vi "mqttCmdAcknowledge.vi"(0 "_mqtt in":refnum<class "mqttCmdPublish.lvclass">, 11 "error in (no error)":errorcluster) -> (4 "_mqtt out":refnum<class "mqttCmdPublish.lvclass">, 8 "notification":T1, 15 "error out":errorcluster)   [LabVIEW 2017, in "mqttCmdPublish.lvclass"]
uses:
  mqttCmdPublish.lvclass
  K:/Cutting Technology/1 - In scope projects/AI3568 Catapult Programme 2017-18/5 - Software Files/development/mqtt Folder/src/class/mqtt/mqttCmd/mqttCmd.lvclass
  mqttTypedef/mqttRXdataCluster.ctl
  mqttTypedef/mqttFixedHeaderResponse.ctl
  mqttTypedef/mqttQOSlevel.ctl
  mqttTypedef/mqttMessageType.ctl
  mqttCmd.lvclass/mqttCmd.ctl
  mqttCmd.lvclass
panel:
  out "timed out? 2":bool
  out "timed out?":bool
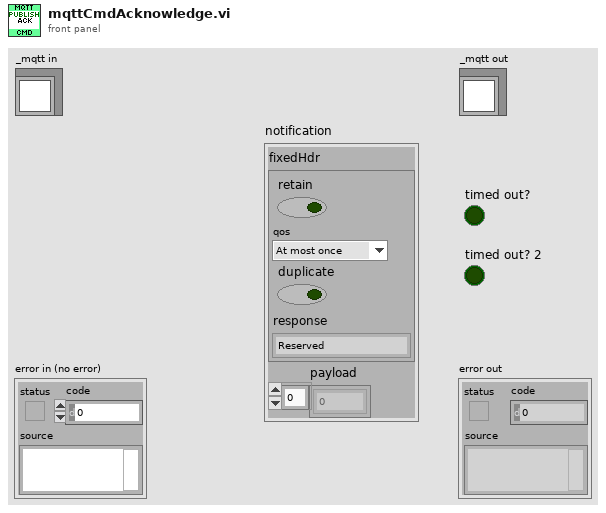
[diagram p1: front panel]
types:
  T1 = typedef "mqttRXdataCluster.ctl" = cluster{"fixedHdr":T2, "payload":u8[]}
  T2 = typedef "mqttFixedHeaderResponse.ctl" = cluster{"retain":bool, "qos":T3, "duplicate":bool, "response":T4}
  T3 = typedef "mqttQOSlevel.ctl" = enum8{"At most once", "At least once", "Exactly once", "Reserved"}
  T4 = typedef "mqttMessageType.ctl" = enum32{"Reserved", "CONNECT", "CONNACK", "PUBLISH", "PUBACK", "PUBREC", "PUBREL", "PUBCOMP", "SUBSCRIBE", "SUBACK", "UNSUBSCRIBE", "UNSUBACK", "PINGREQ", "PINGRESP", "DISCONNECT", "Reserved2"}
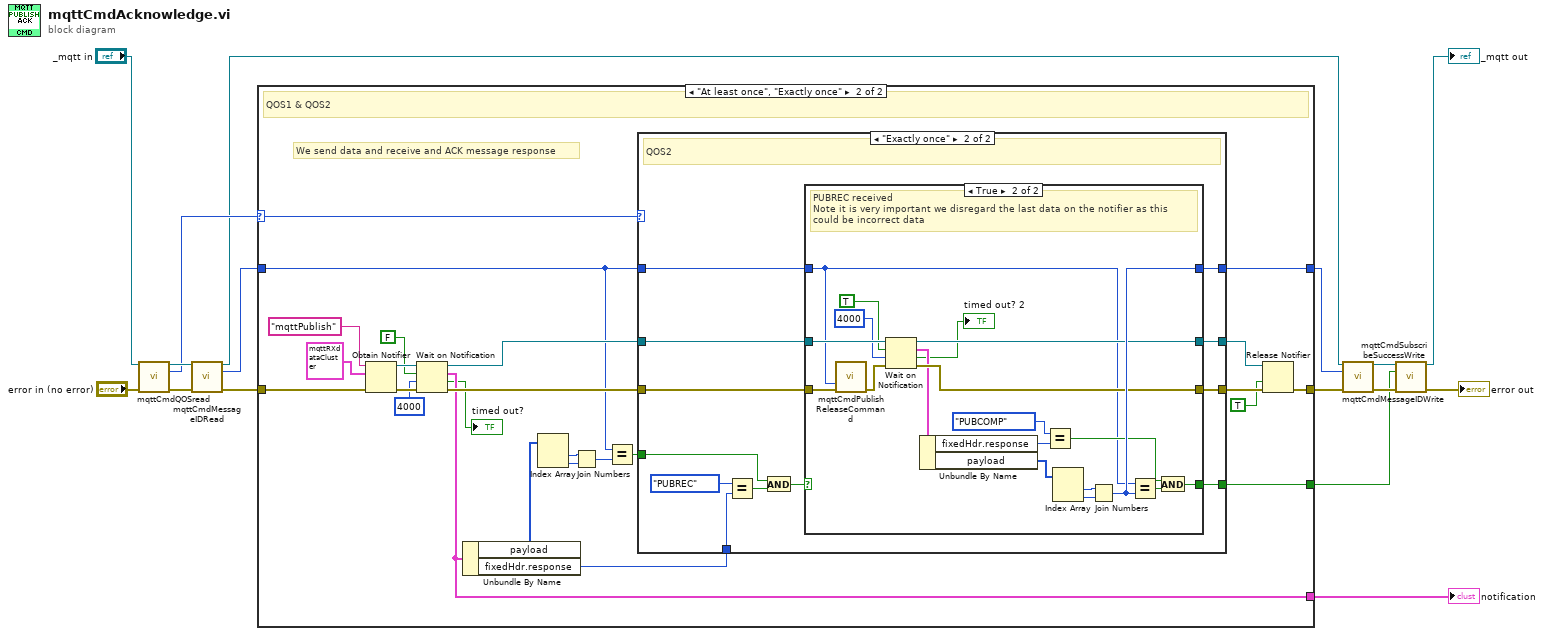
[diagram p0: block diagram]
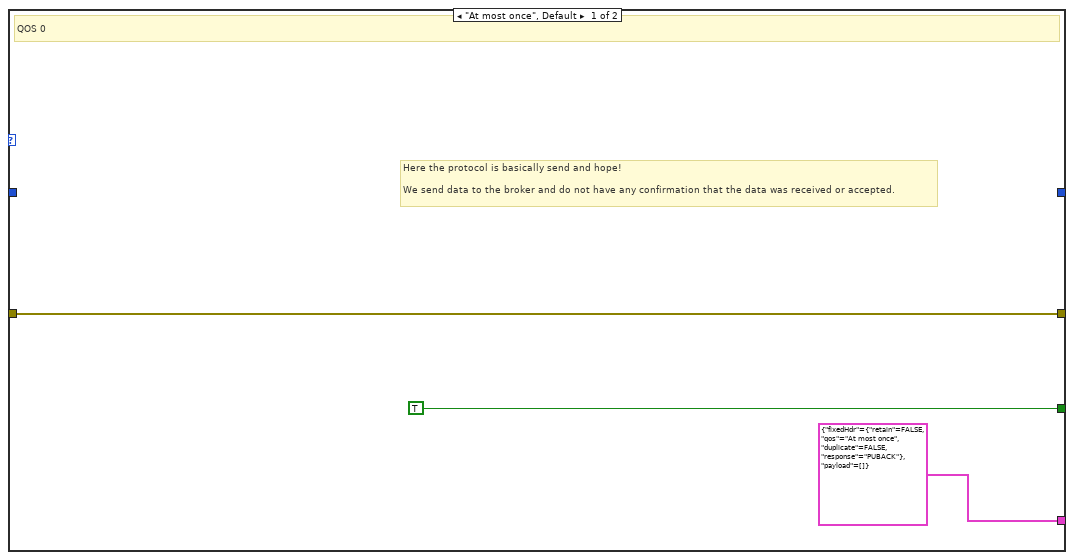
[diagram p2: hidden frame]
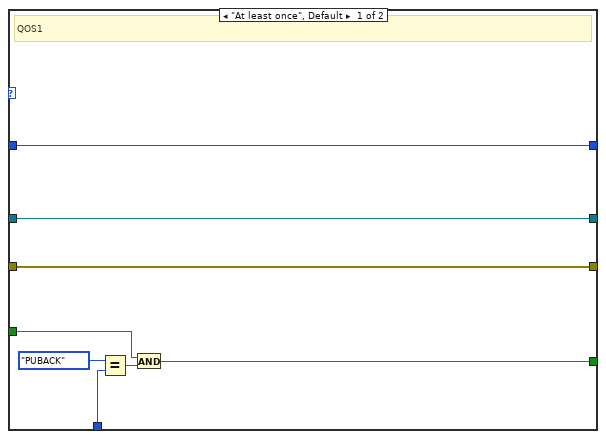
[diagram p3: hidden frame]
diagram:
  n1 = call "mqttCmdQOSread.vi"("mqttBrokerCommand in"="_mqtt in", "error in (no error)"="error in (no error)") -> ("mqttBrokerCommand out"=w14:refnum<class "mqttCmdPublish.lvclass">, "QoS"=w11:T3, "error out"=w15:errorcluster)  [unwired: 11 in]
  n2 = call "mqttCmdMessageIDRead.vi"("mqttBrokerCommand in"=w14, "error in (no error)"=w15) -> ("mqttBrokerCommand out"=w6:refnum<class "mqttCmdPublish.lvclass">, "messageID"=w12:u16, "error out"=w13:errorcluster)  [unwired: 11 in]
  n3 = case shown="\"At least once\", \"Exactly once\"" w11 {
    selector: w11 -> [_ w44]
    tunnel: [w19 w31] -> w9
    tunnel: w13 -> [w19 w38]
    tunnel: [_ w42] -> w8
    tunnel: [TRUE w43] -> w2
    tunnel: w12 -> [_ w25]
    tunnel: [T1 {"fixedHdr"={"retain"=FALSE, "qos"=enum."At most once", "duplicate"=FALSE, "response"=enum."PUBACK"}, "payload"=[]} ("notification") w22] -> w10
    frame "At most once", Default {
      # "Here the protocol is basically send and hope!\n\nWe send data to the broker and do not have any confirmation that the data was received or accepted."
      # "QOS 0"
    }
    frame "At least once", "Exactly once" {
      # "We send data and receive and ACK message response"
      # "QOS1 & QOS2"
      n4 = Obtain Notifier(name (unnamed)="mqttPublish", notification data type=T1 {"fixedHdr"={"retain"=FALSE, "qos"=enum."At most once", "duplicate"=FALSE, "response"=enum."Reserved"}, "payload"=[]} ("notification"), error in (no error)=w38) -> (notifier out=w36:refnum<notifier>, error out=w41:errorcluster)  [unwired: 1 in, 1 out]
      n5 = Wait on Notification(notifier=w36, ignore previous (F)=FALSE, timeout in ms (-1)=4000, error in (no error)=w41) -> (notifier out=w35:refnum<notifier>, notification=w22:T1, timed out?=→"timed out?":bool, error out=w37:errorcluster)
      n6 = Unbundle By Name(w22) -> ("payload"=w27:u8[], "fixedHdr.response"=w23:T4)
      n7 = Index Array(array=w27) -> (element #1=w28:u8, element #2=w29:u8)  [unwired: 2 in]
      n8 = Join Numbers(hi=w28, lo=w29) -> ((hi.lo)=w26:u16)
      n9 = Equal?(x=w25, y=w26) -> (x = y?=w24:bool)
      n10 = case shown="\"Exactly once\"" w44 {
        tunnel: [w45 w62] -> w43
        tunnel: [w52 w64] -> w33
        tunnel: w37 -> [w52 w63]
        tunnel: w25 -> [w48 w54]
        tunnel: [w48 w61] -> w42
        tunnel: w23 -> [w50 w59]
        tunnel: w35 -> [w49 w58]
        tunnel: [w49 w55] -> w34
        tunnel: w24 -> [w47 w53]
        frame "At least once", Default {
          # "QOS1"
          n11 = Equal?(x=mqttMessageType."PUBACK", y=w50) -> (x = y?=w46:bool)
          n12 = And(x=w47, y=w46) -> (x .and. y?=w45:bool)
        }
        frame "Exactly once" {
          # "QOS2"
          n13 = Equal?(x=mqttMessageType."PUBREC", y=w59) -> (x = y?=w57:bool)
          n14 = And(x=w53, y=w57) -> (x .and. y?=w56:bool)
          n15 = case shown="True" w56 {
            selector: w56 -> [w68 _]
            tunnel: [w67 w84] -> w64
            tunnel: w63 -> [w67 w71]
            tunnel: [w68 w87] -> w62
            tunnel: w54 -> [w66 w70]
            tunnel: [w66 w86] -> w61
            tunnel: w58 -> [w65 w85]
            tunnel: [w65 w83] -> w55
            frame False {
            }
            frame True {
              # "PUBREC received\nNote it is very important we disregard the last data on the notifier as this could be incorrect data"
              n16 = call "mqttCmdPublishReleaseCommand.vi"("messageID"=w70, "error in (no error)"=w71) -> ("error out"=w69:errorcluster)  [unwired: 13 in]
              n17 = Wait on Notification(notifier=w85, ignore previous (F)=TRUE, timeout in ms (-1)=4000, error in (no error)=w69) -> (notifier out=w83:refnum<notifier>, notification=w79:T1, timed out?=→"timed out? 2":bool, error out=w84:errorcluster)
              n18 = Unbundle By Name(w79) -> ("fixedHdr.response"=w77:T4, "payload"=w78:u8[])
              n19 = Equal?(x=mqttMessageType."PUBCOMP", y=w77) -> (x = y?=w75:bool)
              n20 = Index Array(array=w78) -> (element #1=w81:u8, element #2=w82:u8)  [unwired: 2 in]
              n21 = Join Numbers(hi=w81, lo=w82) -> ((hi.lo)=w86:u16)
              n22 = Equal?(x=w70, y=w86) -> (x = y?=w74:bool)
              n23 = And(x=w75, y=w74) -> (x .and. y?=w87:bool)
            }
          }
        }
      }
      n24 = Release Notifier(notifier=w34, force destroy? (F)=TRUE, error in (no error)=w33) -> (error out=w31:errorcluster)  [unwired: 2 out]
    }
  }
  "notification" <- w10
  n25 = call "mqttCmdMessageIDWrite.vi"("mqttBrokerCommand in"=w6, "messageID"=w8, "error in (no error)"=w9) -> ("mqttBrokerCommand out"=w3:refnum<class "mqttCmdPublish.lvclass">, "error out"=w5:errorcluster)  [unwired: 11 in]
  n26 = call "mqttCmdSubscribeSuccessWrite.vi"("mqttBrokerCommand in"=w3, "success"=w2, "error in (no error)"=w5) -> ("mqttBrokerCommand out"=→"_mqtt out":refnum<class "mqttCmdPublish.lvclass">, "error out"=→"error out":errorcluster)  [unwired: 11 in]
